vi "Initialize.vi"(8 "error in":errorcluster) -> (0 "error out":errorcluster, 3 "Engine out":refnum<class "Engine.lvclass">)   [LabVIEW 2019, in "Engine.lvclass"]
uses:
  Engine.lvclass
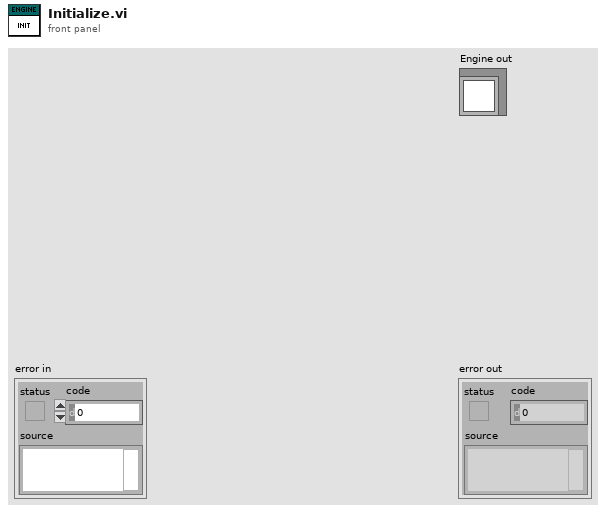
[diagram p1: front panel]
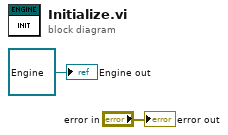
[diagram p0: block diagram]
diagram:
  "error out" <- "error in"
  "Engine out" <- refnum<class "Engine.lvclass"> refnum ("Engine out")
